vi "SendCommand.vi"(7 "Message type":T1="Control", 8 "error in (no error)":errorcluster, 9 "data":variant, 10 "Command":T2="CONTROL:DAQmxConnect", 11 "Control-Client in":refnum<class "Control-Client.lvclass">) -> (0 "error out":errorcluster, 3 "Control-Client out":refnum<class "Control-Client.lvclass">)   [LabVIEW 2018, in "Control-Client.lvclass"]
uses:
  Control-Client.lvclass
  C:/Users/Sergey Denisov/Documents/REPS/TRANCON/Classes/GeneralFunctionality/GeneralFunctionality.lvclass
  dependecies/ControlsVIs/Clusters-def/SERVER-Commands.ctl
  dependecies/ControlsVIs/Clusters-def/Message types.ctl
  Message/Message.lvclass
  GeneralFunctionality/GeneralFunctionality.lvclass
  Control-Server/Control-Server.lvclass
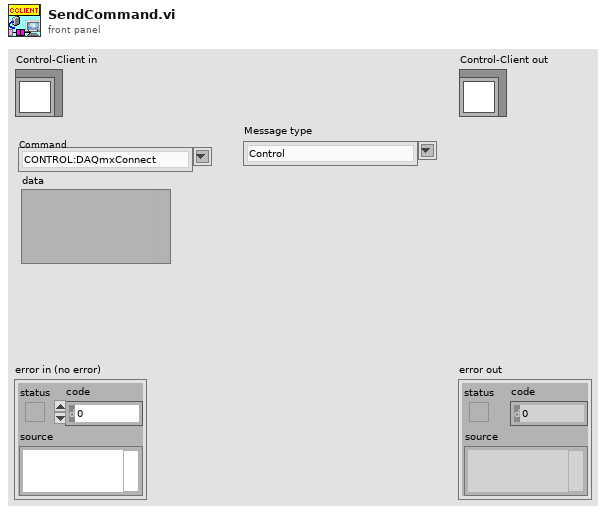
[diagram p1: front panel]
types:
  T1 = typedef "Message types.ctl" = string
  T2 = typedef "Control-Server.lvclass/SERVER-Commands.ctl" = string
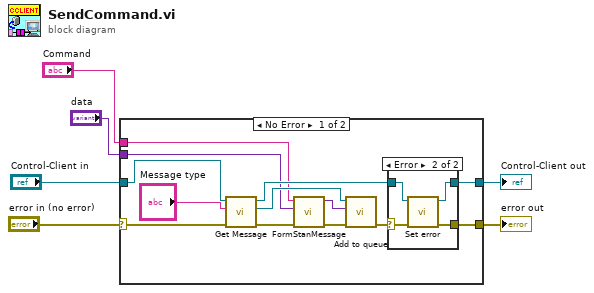
[diagram p0: block diagram]
diagram:
  n1 = case shown="No Error" "error in (no error)" {
    selector: "error in (no error)" -> [w16 w27]
    tunnel: [w13 w27] -> w2
    tunnel: [w14 w26] -> w1
    tunnel: "Control-Client in" -> [w19 w26]
    tunnel: "Command" -> [w9 _]
    tunnel: "data" -> [w8 _]
    frame No Error {
      n2 = call "Get Message.vi"("error in (no error)"=w16, "Message type"="Message type", "GeneralFunctionality en entrée"=w19) -> ("error out"=w12:errorcluster, "Message.lvclass"=w18:refnum<class "Message.lvclass">, "GeneralFunctionality en sortie"=w15:refnum<class "Control-Client.lvclass">)  [unwired: 6 in]
      n3 = call "FormStanMessage.vi"("error in"=w12, "data"=w8, "Command"=w9) -> ("error out"=w11:errorcluster, "message"=w10:variant)  [unwired: 7 in]
      n4 = call "Add to queue.vi"("error in (no error)"=w11, "Data"=w10, "Message in"=w18) -> ("error out"=w7:errorcluster)  [unwired: 7 in, 1 out]
      n5 = case shown="Error" w7 {
        selector: w7 -> [w21 w22]
        tunnel: w15 -> [w20 w25]
        tunnel: [w20 w24] -> w14
        tunnel: [w21 w23] -> w13
        frame No Error {
        }
        frame Error {
          n6 = call "Set error.vi"("error in (no error)"=w22, "Control-Client in"=w25) -> ("error out"=w23:errorcluster, "Control-Client out"=w24:refnum<class "Control-Client.lvclass">)  [unwired: 8 in]
        }
      }
    }
    frame Error {
    }
  }
  "error out" <- w2
  "Control-Client out" <- w1
